vi "Get NVMEM Area Property.vi"   [LabVIEW 2020, in "SLSC.lvlib"]
uses:
  <vilib>/SLSC/SLSC.lvlib
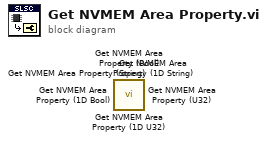
[diagram p0: block diagram]
diagram:
  n1 = call <vilib>:"Get NVMEM Area Property (1D U32).vi"() -> ()  [unwired: 13 in, 3 out]
  n2 = call <vilib>:"Get NVMEM Area Property (1D String).vi"() -> ()  [unwired: 13 in, 3 out]
  n3 = call <vilib>:"Get NVMEM Area Property (1D Bool).vi"() -> ()  [unwired: 13 in, 3 out]
  n4 = call <vilib>:"Get NVMEM Area Property (U32).vi"() -> ()  [unwired: 13 in, 3 out]
  n5 = call <vilib>:"Get NVMEM Area Property (String).vi"() -> ()  [unwired: 13 in, 3 out]
  n6 = call <vilib>:"Get NVMEM Area Property (Bool).vi"() -> ()  [unwired: 13 in, 3 out]
